vi "Symphony ReadTemp.vi"(7 "error in (no error)":errorcluster, 8 "units":u16(ring) items=["° Celsius", "Kelvin", "° Farenheit"], 10 "JYCCDLib.IJYCCDReqd":refnum<k7>) -> (0 "error out":errorcluster, 1 "AcqTime":u32, 2 "Current Temperature":dbl format="%.2f", 3 "reference out":refnum<k7>)   [LabVIEW 2012]
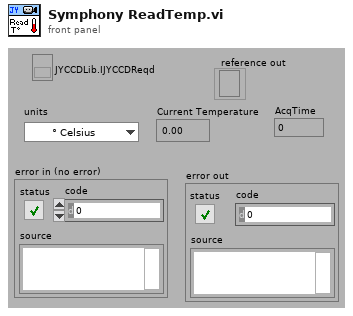
[diagram p1: front panel]
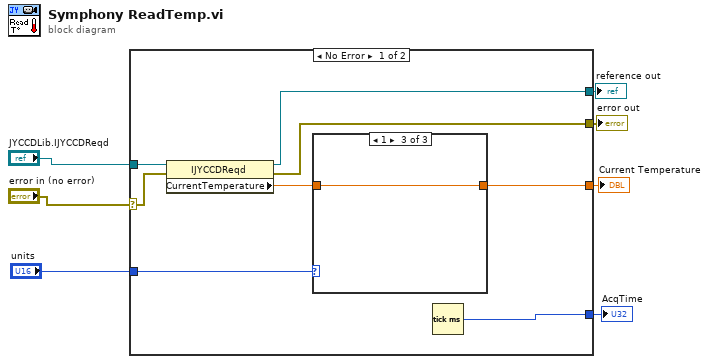
[diagram p0: block diagram]
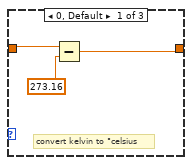
[diagram p2: hidden frame]
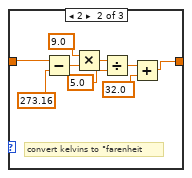
[diagram p3: hidden frame]
diagram:
  n1 = case shown="No Error" "error in (no error)" {
    selector: "error in (no error)" -> [w10 w30]
    tunnel: "JYCCDLib.IJYCCDReqd" -> [w15 w29]
    tunnel: "units" -> [w14 _]
    tunnel: [w12 _] -> w5
    tunnel: [w11 w29] -> w4
    tunnel: [w9 w30] -> w2
    tunnel: [w8 _] -> w1
    frame No Error {
      n2 = property class="IJYCCDReqd"(reference=w15, error in=w10) -> (reference out=w11:refnum<k7>, error out=w9:errorcluster, "CurrentTemperature"=w13:dbl)
      n3 = case shown="1" w14 {
        tunnel: w13 -> [w18 w27 w28]
        tunnel: [w16 w19 w28] -> w12
        frame 0, Default {
          # "convert kelvin to °celsius"
          n4 = Subtract(x=w18, y=273.16) -> (x-y=w16:dbl)
        }
        frame 2 {
          # "convert kelvins to °farenheit"
          n5 = Subtract(x=w27, y=273.16) -> (x-y=w25:dbl)
          n6 = Multiply(x=9.0, y=w25) -> (x*y=w23:dbl)
          n7 = Divide(x=w23, y=5.0) -> (x/y=w21:dbl)
          n8 = Add(x=w21, y=32.0) -> (x+y=w19:dbl)
        }
        frame 1 {
        }
      }
      n9 = Tick Count (ms)() -> (millisecond timer value=w8:u32)
    }
    frame Error {
    }
  }
  "Current Temperature" <- w5
  "reference out" <- w4
  "error out" <- w2
  "AcqTime" <- w1
